vi "subVI_close3CONEXactuators.vi"(3 "error in (no error)":errorcluster, 5 "CONEX Cluster":T1) -> (0 "Error OUT":errorcluster)   [LabVIEW 2010]
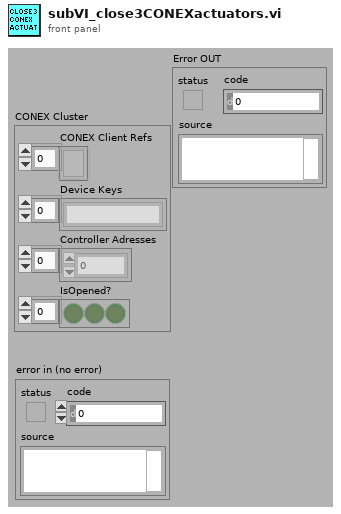
[diagram p1: front panel]
types:
  T1 = cluster{"CONEX Client Refs":refnum<k24>[], "Device Keys":string[], "Controller Adresses":i32[], "IsOpened?":bool[]}
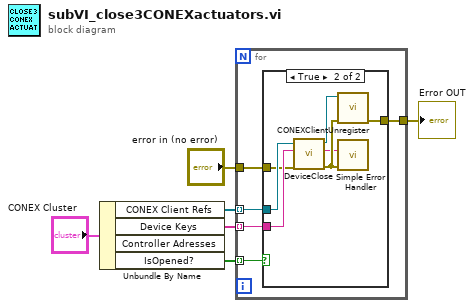
[diagram p0: block diagram]
diagram:
  n1 = Unbundle By Name("CONEX Cluster") -> ("CONEX Client Refs"=w6:refnum<k24>[], "Device Keys"=w5:string[], "IsOpened?"=w1:bool[])  [unwired: 1 out]
  n2 = for {
    tunnel: w6 -> [w11] mode=indexing
    tunnel: w5 -> [w10] mode=indexing
    tunnel: "error in (no error)" -> [w9]
    tunnel: [w8] -> w2
    tunnel: w1 -> [w7] mode=indexing
    n3 = case shown="True" w7 {
      tunnel: w11 -> [_ w16]
      tunnel: w10 -> [_ w15]
      tunnel: w9 -> [w12 w14]
      tunnel: [w12 w19] -> w8
      frame False {
      }
      frame True {
        n4 = call <userlib>:"DeviceClose.vi"("Error IN"=w14, "deviceKey IN"=w15, "CONEX Client Ref IN"=w16) -> ("Error OUT"=w18:errorcluster, "deviceKey OUT"=w17:string, "CONEX Client Ref OUT"=w13:refnum<k24>)  [unwired: 6 in]
        n5 = call <userlib>:"CONEXClientUnregister.vi"("Error IN"=w18, "CONEX Client Ref IN"=w13) -> ("Error OUT"=w19:errorcluster)  [unwired: 9 out]
        n6 = call <vilib>:"Simple Error Handler.vi"("error source (\" \")"=w17, "error in (no error)"=w18) -> ()  [unwired: 1 in, 7 out]
      }
    }
  }
  "Error OUT" <- w2
